vi "DirettoreInitMatrix.vi"(10 "dimension size":i32=16, 11 "matrix length in":i32=65535) -> (3 "matrix bank":i32[][](array[numeric]))   [LabVIEW 2012]
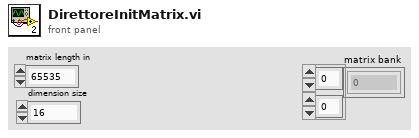
[diagram p1: front panel]
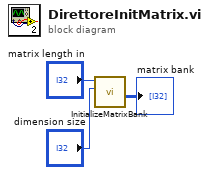
[diagram p0: block diagram]
diagram:
  n1 = call "InitializeMatrixBank.vi"("dimension size"="dimension size", "matrix length in"="matrix length in") -> ("matrix bank"=→"matrix bank":i32[][])  [unwired: 8 in, 1 out]
